vi "Get Description.vi"(8 "error in (no error)":errorcluster, 11 "CIPC Reference":u64) -> (0 "error out":errorcluster, 3 "Description":string)   [LabVIEW 2021, in "CIF_NI_CIPC.lvlib"]
uses:
  CIF_NI_CIPC.lvlib
  libnicipc.dll
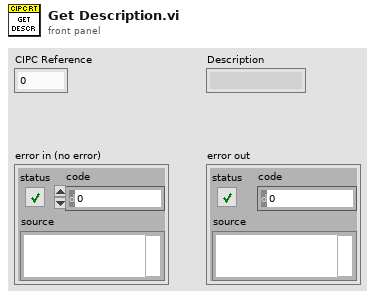
[diagram p1: front panel]
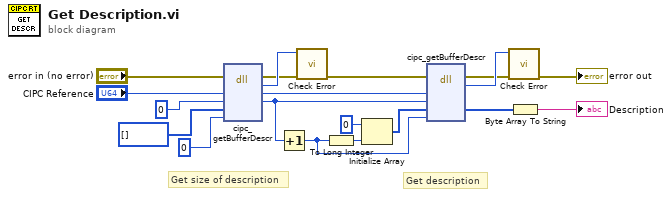
[diagram p0: block diagram]
diagram:
  # "Get description"
  # "Get size of description"
  n1 = dll-call lib="libnicipc.*" fn="cipc_getBufferDescr"(error in="error in (no error)", "cipc_buffer_ref"="CIPC Reference", "descr_size"=u32 0, "el_descr"=u8[] [] ("initialized array"), "el_descr_maxsize"=u32 0) -> (error out=w18:errorcluster, "return type"=w19:i32, "cipc_buffer_ref"=w14:u64, "descr_size"=w10:u32)  [unwired: 4 in, 1 out]
  n2 = Increment(x=w10) -> (x+1=w9:u32)
  n3 = call "Check Error.vi"("error in (no error)"=w18, "Error Code"=w19) -> ("error out"=w15:errorcluster)  [unwired: 9 in]
  n4 = To Long Integer(number=w9) -> (32bit integer=w1:i32)
  n5 = Initialize Array(u8 0, w1) -> (w6:u8[])
  n6 = dll-call lib="libnicipc.*" fn="cipc_getBufferDescr"(error in=w15, "cipc_buffer_ref"=w14, "descr_size"=w10, "el_descr"=w6, "el_descr_maxsize"=w9) -> (error out=w16:errorcluster, "return type"=w17:i32, "el_descr"=w8:u8[])  [unwired: 5 in, 1 out]
  n7 = call "Check Error.vi"("error in (no error)"=w16, "Error Code"=w17) -> ("error out"=→"error out":errorcluster)  [unwired: 9 in]
  n8 = Byte Array To String(unsigned byte array=w8) -> (string=→"Description":string)
